vi "Sequence setup GUI.vi"(11 "error in (no error)":errorcluster) -> (8 "OK":bool, 15 "error out":errorcluster)   [LabVIEW 2011]
uses:
  Sequence step GUI.ctl
  X-cont Action select/Action select.xctl
  X-cont criteria/Criteria control.xctl
  Boolean operation.ctl
  User input.ctl
  Complete sequence cluster holder.ctl
  Sequence steps config..ctl
  Single criteria cluster.ctl
  Criteria types.ctl
panel:
  in  "User input 1":T1={"Input name"="", "Minimum value "=-inf, "Maximum value"=inf, "Default value"=0.0, "User inp enabled"=FALSE}
  in  "Move up":bool
  in  "Move down":bool
  in  "Sequences":i32(listbox)
  in  "Delete step":bool
  in  "Add step":bool
  in  "Delete sequence":bool
  in  "New sequence":bool
  in  "Step":T2
  in  "Steps":i32(listbox)
  out "Mode":bool
  in  "Help":bool
  in  "Done":bool
  # "User input"
  # "Tab header s can be changed as wanted\n\nCustom can be used for completly ccutom behavior,\nmust then highjack  an other hidden page, for settings"
  # "Add custom behavior taht cvan not be replicated by a simple cluster with valisdity checking"
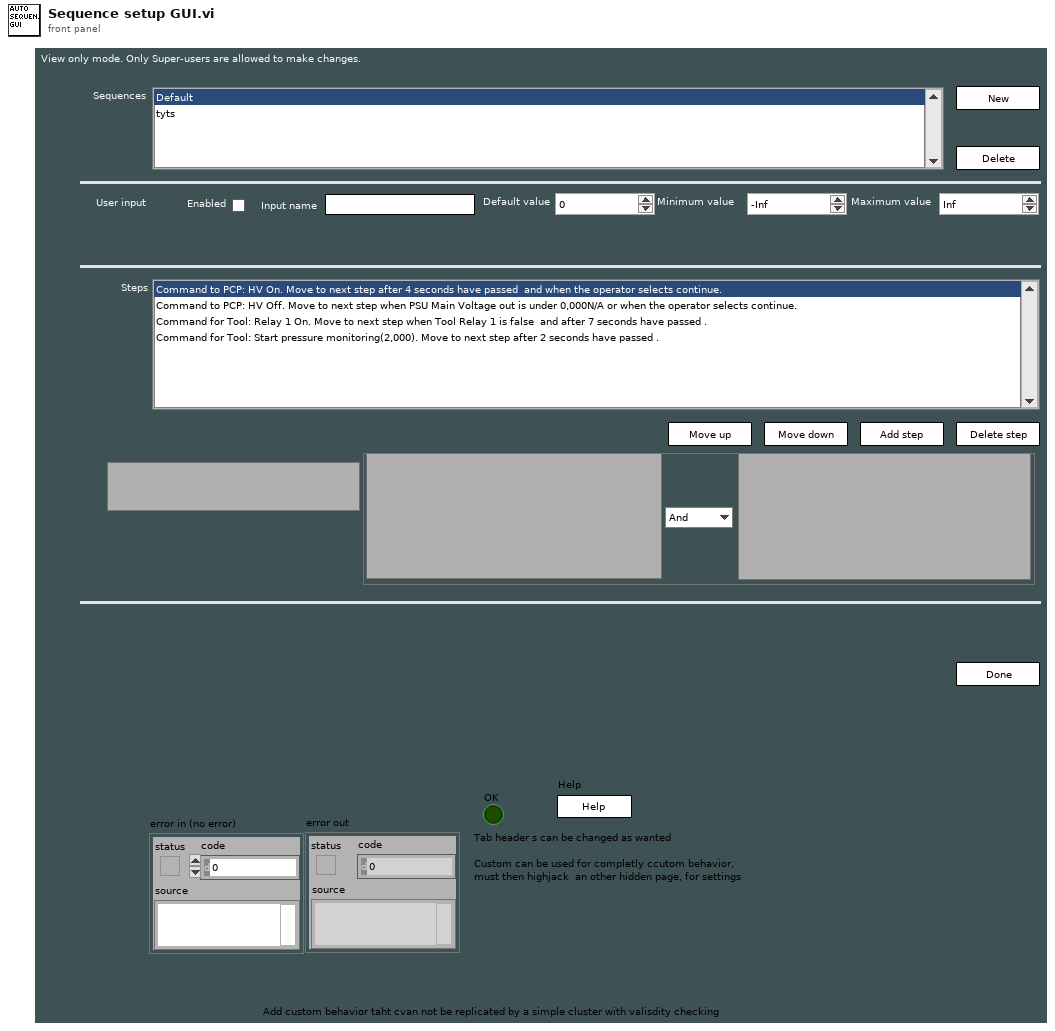
[diagram p1: front panel]
types:
  T1 = typedef "User input.ctl" = cluster{"Input name":string, "Minimum value ":dbl, "Maximum value":dbl, "Default value":dbl, "User inp enabled":bool}
  T2 = typedef "Sequence step GUI.ctl" = cluster{"Action select":cluster{"Action index":i32, "Data":dbl}, "Criteria 1":cluster{"Criteria":T3}, "C1 op C2":T5, "Criteria 2":cluster{"Criteria":T3}}
  T3 = typedef "Single criteria cluster.ctl" = cluster{"Criteria":T4, "Time or analog value":dbl, "Primary IO index":i32, "Secondary  IO index":i32, "User_input":bool}
  T4 = typedef "Criteria types.ctl" = enum16{"No criteria(True)", "Time(s)", "Analog IO over", "Analog IO over or equal", "Analog IO under", "Analog IO under or equal", "Analog IO 1 minus Analog IO 2 over", "Digital IO True", "Digital IO False", "Operator approval"}
  T5 = typedef "Boolean operation.ctl" = enum16{"And", "Or", "Xor", "Nand", "Nor", "Nxor", "Implies"}
  T6 = enum16{"GET", "SET", "Get from Ini", "Put in Ini"}
  T7 = typedef "User Indikator.ctl" = cluster{"User Name":string, "Super User":T8}
  T8 = typedef "Super User bool indikator.ctl" = bool
  T9 = enum8{"Enabled", "Disabled", "Disabled and Grayed Out"}
  T10 = typedef "Sequence steps config..ctl" = cluster{"Enabled":bool, "Criteria 1":T3, "C1 op C2":T5, "Criteria 2":T3, "Action index":i32, "Action Name":string, "Action value":dbl}
  T11 = typedef "Fixed Analog Channel Definition.ctl" = cluster{"ID":u16, "Name":string, "Quantity":T12, "Unit":string, "Maximum upd":T13, "Comment":string, "Help file Name":string, "Help file Section ":string, "Category":T14, "User adjustable Scaling":bool, "Default Scaling":T15, "Default Unit":i32, "Classification":T16}
  T12 = typedef "Quantity enum.ctl" = enum16{"NA", "Acceleration", "Angle", "Current", "Force", "Distance", "Pressure", "Resistance", "Rotational Speed", "Speed", "Temperature", "Tension", "Torque", "Voltage", "Weight"}
  T13 = typedef "Update frequensies.ctl" = enum16{"2 Hz", "1 Hz", "0.1 Hz"}
  T14 = typedef "Channel catagory Enum.ctl" = enum16{"No Category", "Power", "Temperature", "Pressure"}
  T15 = typedef "Scaling.ctl" = cluster{"Gain":dbl, "Offset":dbl}
  T16 = typedef "Channel Classification Enum.ctl" = enum16{"Basic", "Advanced", "Expert", "Unused"}
  T17 = typedef "Fixed Digital Channel Definition.ctl" = cluster{"ID":u16, "Name":string, "NA Text":string, "Off Text":string, "On Text":string, "Maximum upd":T13, "Comment":string, "Help file Name":string, "Help file Section ":string, "Catagory":T14, "In use":bool}
  T18 = typedef "Analog Var Disp 0 sif.ctl" = cluster{"Value":dbl, "Unit":string, "Status":T19}
  T19 = typedef "Status indicator Black Small.ctl" = u16
  T20 = typedef "Action colleciton cluster.ctl" = cluster{"common":T21, "Action type":T23, "General command":T24, "PCP command":T25, "Tool command":T26}
  T21 = typedef "Action common elements.ctl" = cluster{"Name":string, "Adjuster type":T22, "Adjuster double default value":dbl}
  T22 = typedef "Action adjuster type.ctl" = enum16{"Non", "Double"}
  T23 = typedef "Action type.ctl" = enum16{"General", "PCP command", "Tool command"}
  T24 = typedef "General command list.ctl" = enum16{"No action"}
  T25 = typedef "PCP High Level Commands.ctl" = enum16{"HVPSU HV ON", "HVPSU HV OFF", "PCP PC", "PCP Local", "Update Motor Voltage", "Update Cable Resistance", "Final Motor Voltage", "Final Resistance"}
  T26 = typedef "Tool specific commands.ctl" = enum16{"controller relay 1 on", "controller relay 1 off", "controller relay 2 on", "controller relay 2 off", "Solonoid 1 (master) on", "Solonoid 1 (master) off", "Solonoid 2 (Stroker) on", "Solonoid 2 (Stroker) off", "Solonoid 3 (Anchor) on", "Solonoid 3 (Anchor) off", "Controller relay 1 & 2 on", "Controller relay 1 & 2 off", "Controller relay 1 on, 2 off", "Controller relay 1 off, 2 on", "STROKER tool: Stop Force Mon", "High-G Stop", "High-G Get data", "High-G Stop Get data", "STROKER tool: Stroke out", "STROKER tool: Stroke in", "STROKER tool: Stroke stop", "STROKER tool: Stroke go to", "STROKER tool: Stop Homing", "STROKER tool: Start Force Mon dir in", "STROKER tool: Start Force Mon dir out", "Controller STOP"}
  T27 = typedef "Complete sequence cluster holder.ctl" = cluster{"Sequence Name":string, "User input 1":T1, "Steps":T10[]}
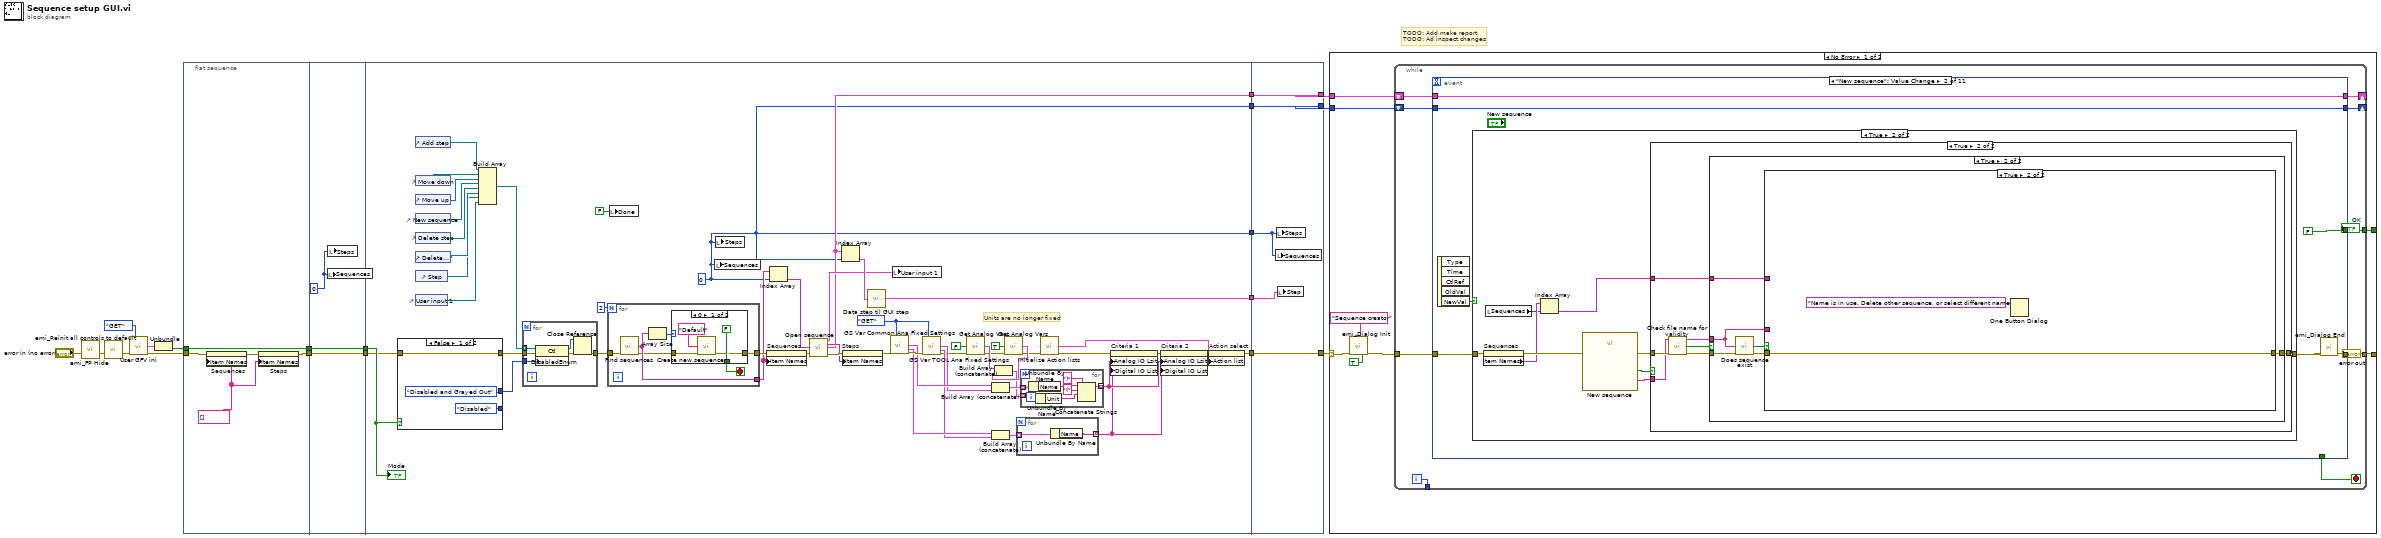
[diagram p0: block diagram]
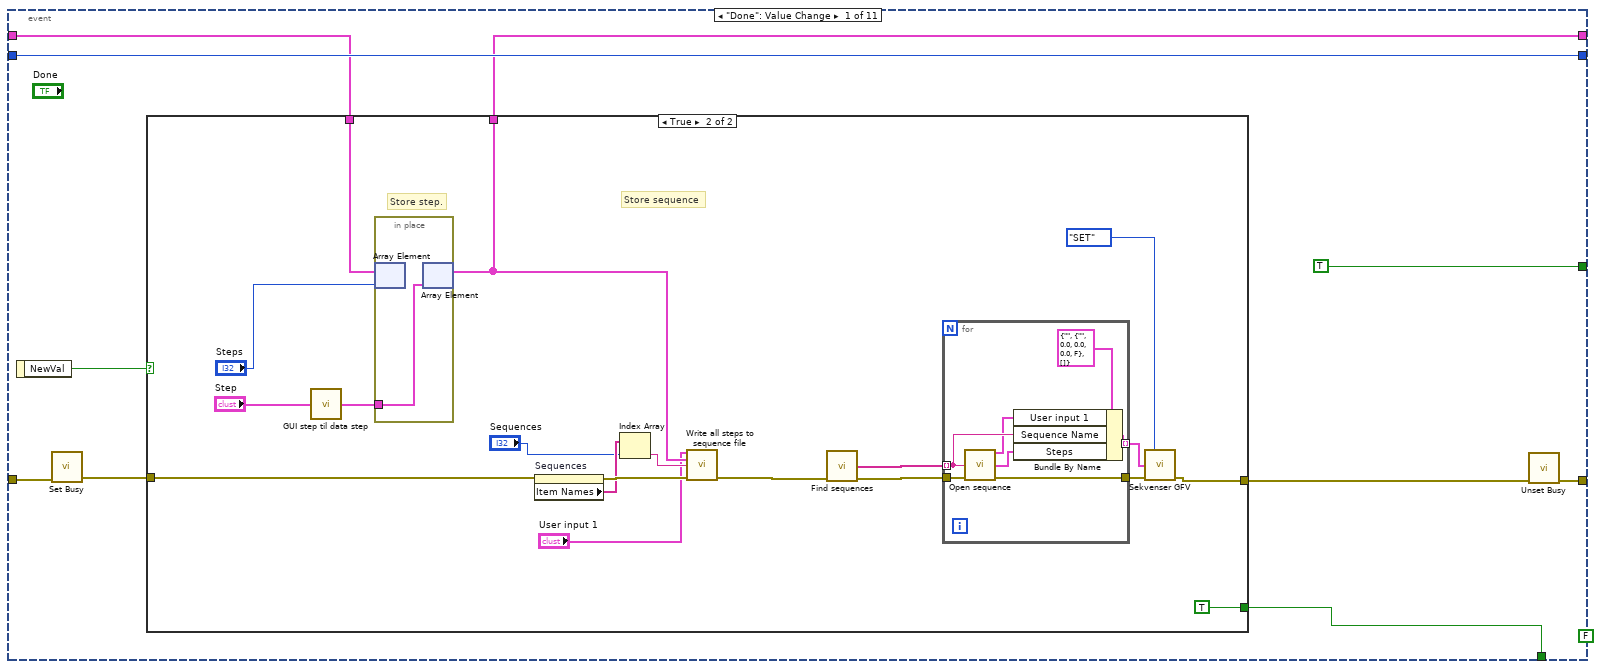
[diagram p2: hidden frame]
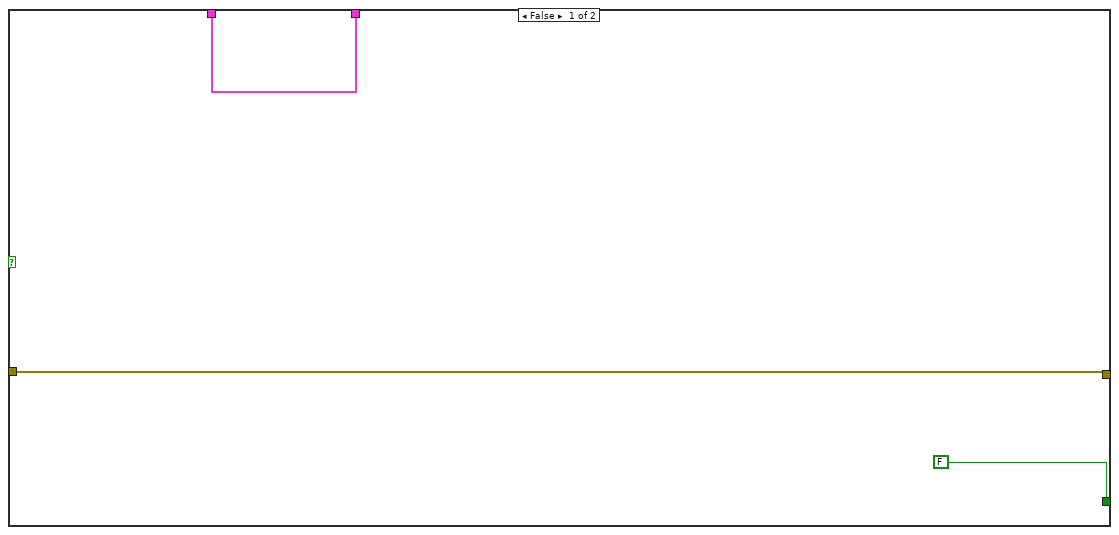
[diagram p3: hidden frame]
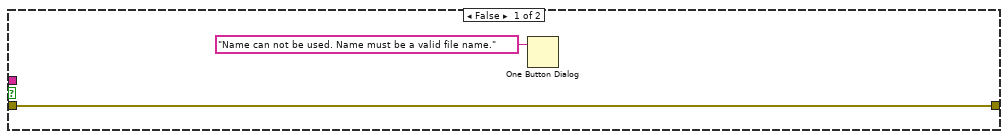
[diagram p6: hidden frame]
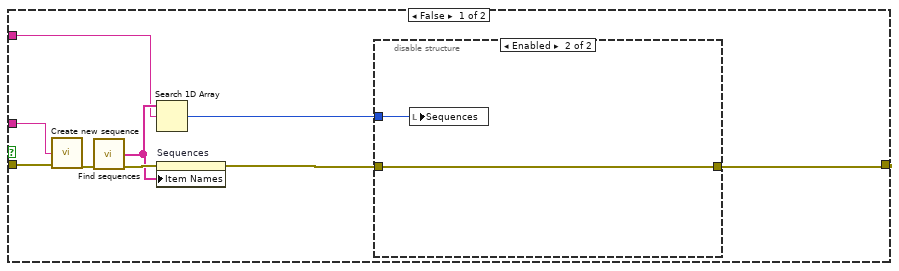
[diagram p7: hidden frame]
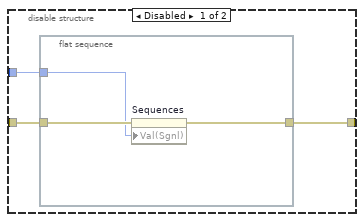
[diagram p8: hidden frame]
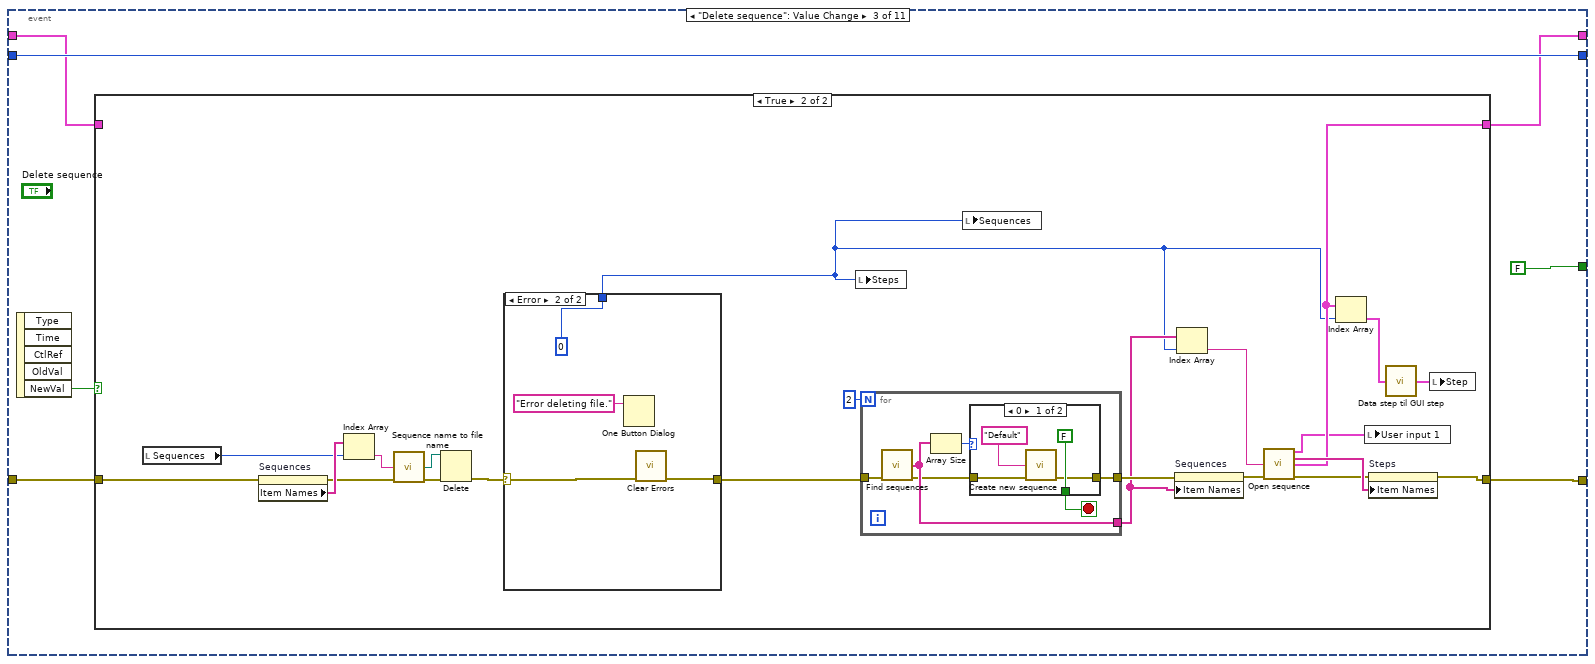
[diagram p9: hidden frame]
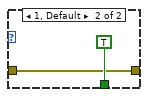
[diagram p11: hidden frame]
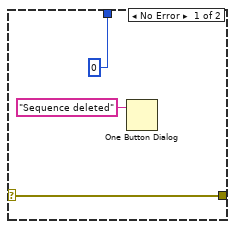
[diagram p12: hidden frame]
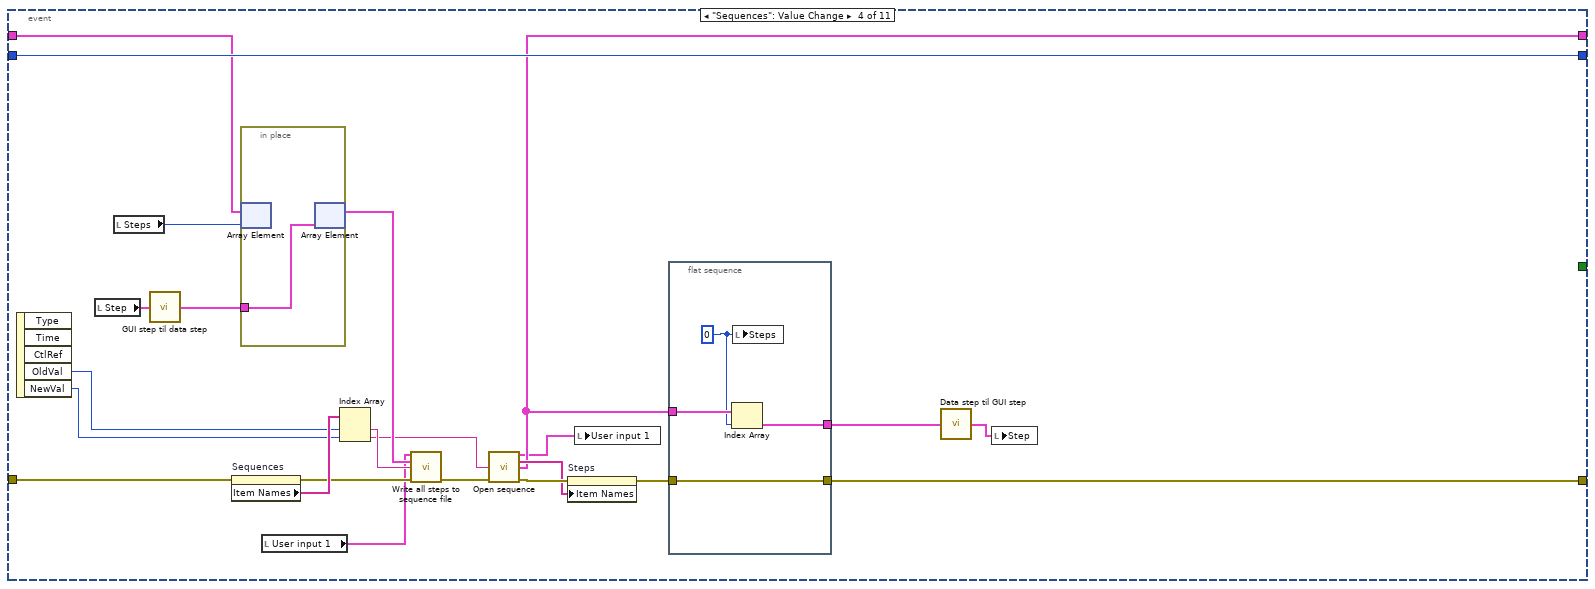
[diagram p13: hidden frame]
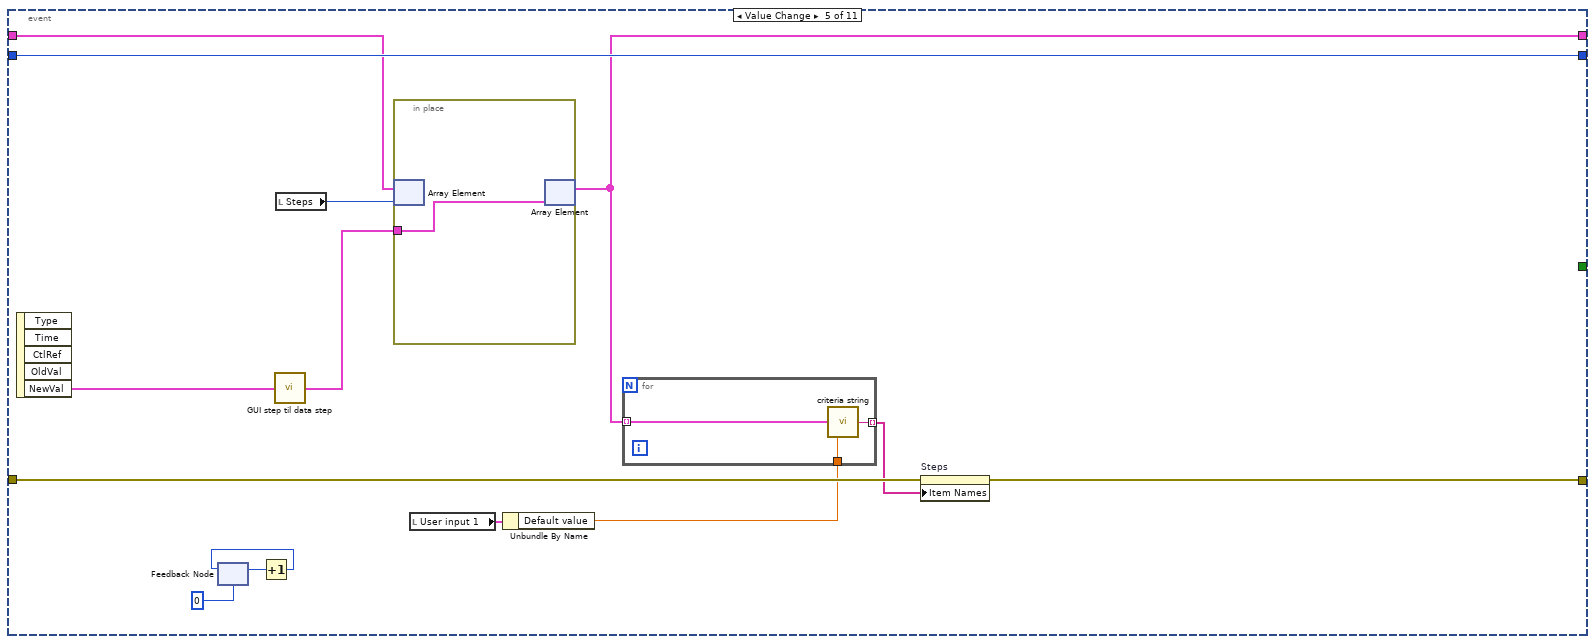
[diagram p14: hidden frame]
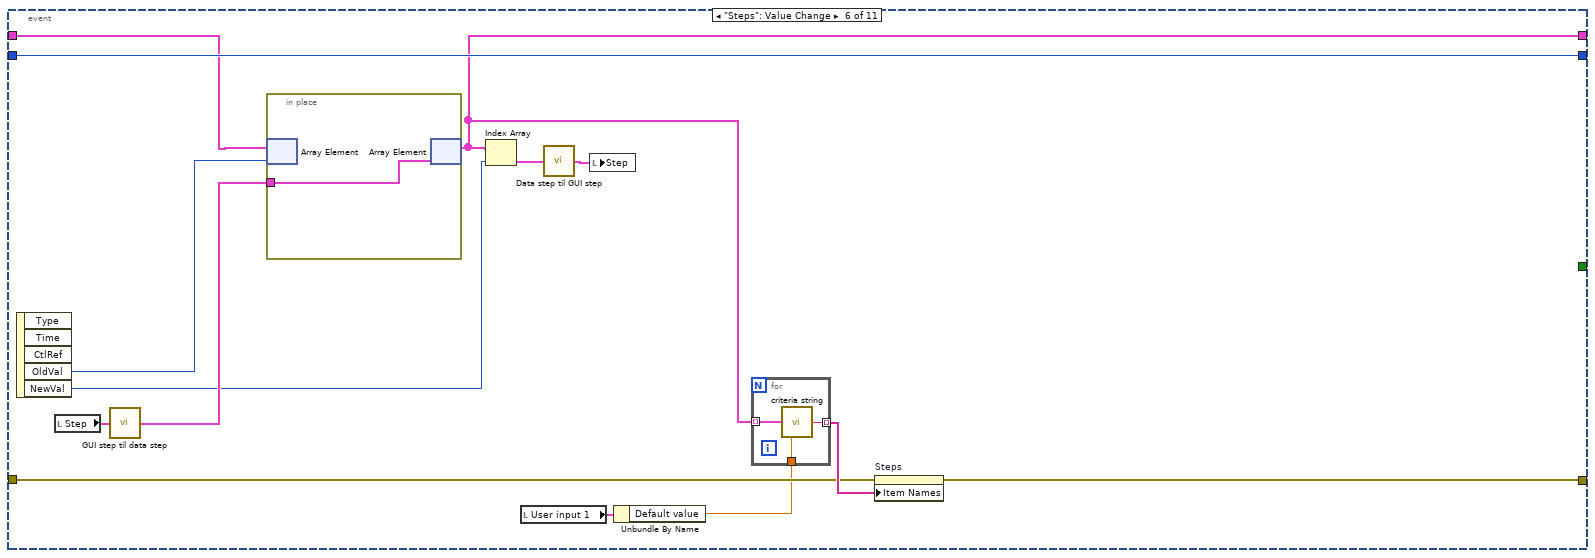
[diagram p15: hidden frame]
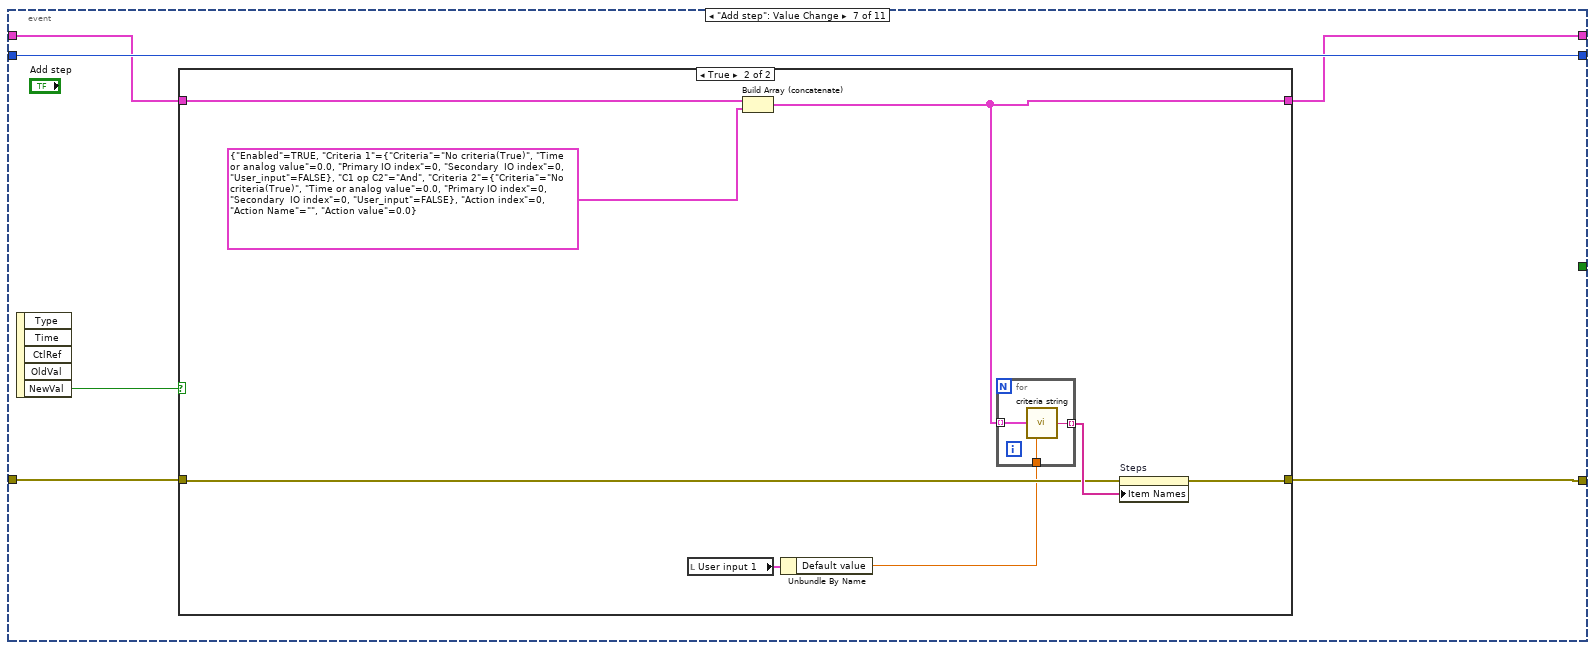
[diagram p16: hidden frame]
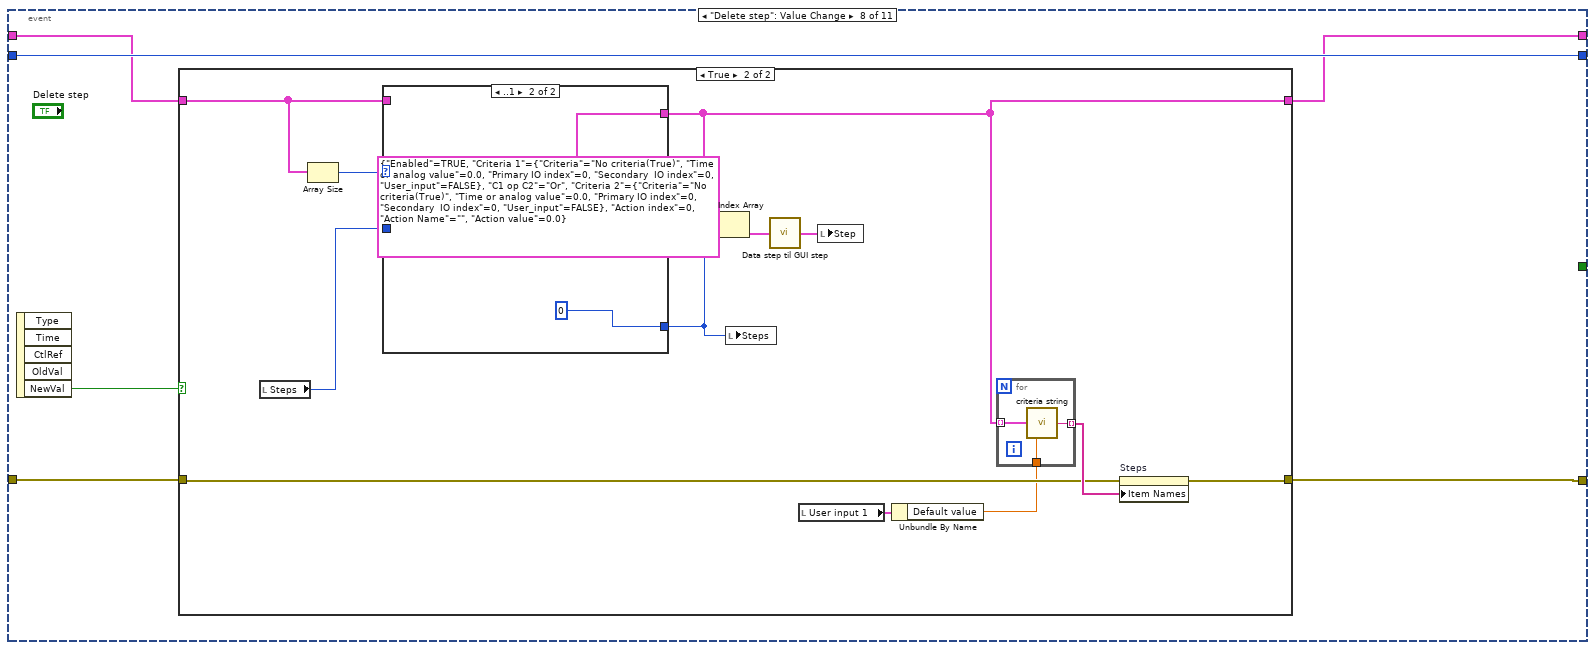
[diagram p18: hidden frame]
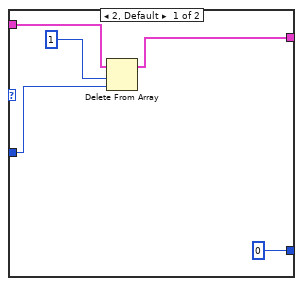
[diagram p20: hidden frame]
diagram:
  # "TODO: Add make report\nTODO: Ad inspect changes"
  n1 = call "emi_FP Hide.vi"("error in (no error)"="error in (no error)") -> ("error out"=w18:errorcluster)  [unwired: 13 in, 1 out]
  n2 = call "emi_Reinit all controls to default.vi"("error in (no error)"=w18) -> ("error out"=w16:errorcluster)  [unwired: 13 in, 1 out]
  n3 = call "User GFV ini.vi"("Action(GET)"=T6."GET", "error in (no error)"=w16) -> ("User ID out"=w15:T7, "error out"=w14:errorcluster)  [unwired: 12 in]
  n4 = Unbundle(w15) -> ("Super User"=w13:T8)  [unwired: 1 out]
  n5 = flat-sequence {
    tunnel: w13 -> [w27]
    tunnel: w14 -> [w26]
    tunnel: [w23] -> w9
    tunnel: [w27] -> w7
    tunnel: w9 -> [w30]
    tunnel: [w30] -> w8
    tunnel: w7 -> [w29]
    tunnel: [w29] -> w6
    tunnel: w8 -> [w80]
    tunnel: w6 -> [w81]
    tunnel: [w47] -> w5
    tunnel: [w42] -> w4
    tunnel: [w41] -> w3
    tunnel: [w41] -> w2
    tunnel: [w40] -> w1
    tunnel: [w116] -> w10
    tunnel: [w117] -> w11
    tunnel: [w118] -> w17
    tunnel: w5 -> [w118]
    tunnel: w4 -> [w117]
    tunnel: w3 -> [w116]
    tunnel: w2 -> [w115]
    tunnel: w1 -> [w114]
    frame #0 {
      w24 = string[] [] ("Item Names")
      n6 = property on="Sequences" class="LstBox (strict)"(error in=w26, "Item Names"=w24) -> (error out=w25:errorcluster)  [unwired: 1 in, 1 out]
      n7 = property on="Steps" class="LstBox (strict)"(error in=w25, "Item Names"=w24) -> (error out=w23:errorcluster)  [unwired: 1 in, 1 out]
    }
    frame #1 {
      w28 = 0 ("Sequences")
      n8 = local write "Sequences"(w28) -> ()
      n9 = local write "Steps"(w28) -> ()
    }
    frame #2 {
      w59 = enum16{"GET", "SET"}."GET" ("Action(GET)")
      w41 = 0 ("Sequences")
      # "Units are no longer fixed"
      n10 = case shown="False" w81 {
        tunnel: w80 -> [w110 w113]
        tunnel: [w110 w113] -> w65
        tunnel: [T9."Disabled and Grayed Out" ("Disabled") w112] -> w61
        tunnel: [T9."Disabled" ("Disabled") w112] -> _
        frame False {
        }
        frame True {
          w112 = T9."Enabled" ("Disabled")
        }
      }
      n11 = control-ref of="Add step"() -> (w66:refnum<vi>)
      n12 = control-ref of="Move down"() -> (w67:refnum<vi>)
      n13 = control-ref of="Move up"() -> (w68:refnum<vi>)
      n14 = control-ref of="New sequence"() -> (w69:refnum<vi>)
      n15 = control-ref of="Delete step"() -> (w70:refnum<vi>)
      n16 = control-ref of="Delete sequence"() -> (w71:refnum<vi>)
      n17 = control-ref of="Step"() -> (w62:refnum<vi>)
      n18 = control-ref of="User input 1"() -> (w43:refnum<vi>)
      n19 = Build Array(w66, w67, w68, w69, w70, w71, w62, w43) -> (w63:refnum<vi>[])
      n20 = for {
        tunnel: w65 -> [w96]
        tunnel: [w94] -> w64
        tunnel: w63 -> [w92] mode=indexing
        tunnel: w61 -> [w91]
        n21 = property class="Ctl"(reference=w92, error in=w96, "DisabledEnum"=w91) -> (reference out=w93:refnum<vi>, error out=w95:errorcluster)
        n22 = Close Reference(reference=w93, error in (no error)=w95) -> (error out=w94:errorcluster)
      }
      n23 = for {
        N: 2 -> [_]
        tunnel: w64 -> [w102]
        tunnel: [w97] -> w79
        tunnel: [w101] -> w77
        stop <- w98 stop-if-true
        n24 = call "Find sequences.vi"("error in (no error)"=w102) -> ("Sequences"=w101:string[], "error out"=w100:errorcluster)  [unwired: 13 in]
        n25 = Array Size(array=w101) -> (size(s)=w99:i32)
        n26 = case shown="0" w99 {
          tunnel: w100 -> [w105 w107]
          tunnel: [FALSE TRUE] -> w98
          tunnel: [w104 w107] -> w97
          frame 0 {
            n27 = call "Create new sequence.vi"("Sequence name"="Default", "error in (no error)"=w105) -> ("error out"=w104:errorcluster)  [unwired: 13 in]
          }
          frame 1, Default {
          }
        }
      }
      n28 = local write "Done"(FALSE ("Done")) -> ()
      n29 = local write "Sequences"(w41) -> ()
      n30 = local write "Steps"(w41) -> ()
      n31 = property on="Sequences" class="LstBox (strict)"(error in=w79, "Item Names"=w77) -> (error out=w76:errorcluster)  [unwired: 1 in, 1 out]
      n32 = Index Array(array=w77, index=w41) -> (element=w75:string)
      n33 = call "Open sequence.vi"("Sequence name"=w75, "error in (no error)"=w76) -> ("User input 1"=w44:T1, "string steps"=w73:string[], "Steps"=w42:T10[], "error out"=w74:errorcluster)  [unwired: 9 in, 1 out]
      n34 = Index Array(array=w42, index=w41) -> (element=w72:T10)
      n35 = property on="Steps" class="LstBox (strict)"(error in=w74, "Item Names"=w73) -> (error out=w52:errorcluster)  [unwired: 1 in, 1 out]
      n36 = call "Data step til GUI step.vi"("data step cluster"=w72) -> ("GUI step clluster"=w40:T2)  [unwired: 13 in, 1 out]
      n37 = call "GS Var Common Ana Fixed Settings.vi"("Action(GET)"=w59, "error in (no error)"=w52) -> ("Common Analog Var Fixed out"=w58:T11[], "Common Digital var Fixed"=w56:T17[], "error out"=w60:errorcluster)  [unwired: 11 in]
      n38 = local write "User input 1"(w44) -> ()
      n39 = call "GS Var TOOL Ana Fixed Settings.vi"("Action(GET)"=w59, "error in (no error)"=w60) -> ("Tool Analog var Fixed out"=w57:T11[], "Tool Digital Var Fixed out"=w55:T17[], "error out"=w34:errorcluster)  [unwired: 11 in]
      n40 = call "Get Analog Vars.vi"("Tool"=FALSE, "error in (no error)"=w34) -> ("Analog Vars"=w38:T18[], "error out"=w37:errorcluster)  [unwired: 7 in, 5 out]
      n41 = Build Array (concatenate)(w58, w57) -> (w54:T11[])
      n42 = Build Array (concatenate)(w56, w55) -> (w53:T17[])
      n43 = call "Get Analog Vars.vi"("Tool"=TRUE, "error in (no error)"=w37) -> ("Analog Vars"=w39:T18[], "error out"=w33:errorcluster)  [unwired: 7 in, 5 out]
      n44 = Build Array (concatenate)(w38, w39) -> (w31:T18[])
      n45 = for {
        tunnel: w53 -> [w83] mode=indexing
        tunnel: [w82] -> w49 mode=indexing
        n46 = Unbundle By Name(w83) -> ("Name"=w82:string)
      }
      n47 = for {
        tunnel: w54 -> [w90] mode=indexing
        tunnel: [w88] -> w50 mode=indexing
        tunnel: w31 -> [w85] mode=indexing
        n48 = Unbundle By Name(w90) -> ("Name"=w89:string)
        n49 = Unbundle By Name(w85) -> ("Unit"=w84:string)
        n50 = Concatenate Strings(w89, "(" ("string"), w84, ")" ("string")) -> (w88:string)
      }
      n51 = call "Initialize Action lists.vi"("error in (no error)"=w33) -> ("Actions"=w32:T20[], "error out"=w46:errorcluster)  [unwired: 12 in, 1 out]
      n52 = property on="Criteria 1" class="Criteria control (strict)"(error in=w46, "Analog IO Lsit"=w50, "Digital IO List"=w49) -> (error out=w51:errorcluster)  [unwired: 1 in, 1 out]
      n53 = property on="Criteria 2" class="Criteria control (strict)"(error in=w51, "Analog IO Lsit"=w50, "Digital IO List"=w49) -> (error out=w48:errorcluster)  [unwired: 1 in, 1 out]
      n54 = property on="Action select" class="Action select (strict)"(error in=w48, "Action list"=w32) -> (error out=w47:errorcluster)  [unwired: 1 in, 1 out]
      "Mode" <- w81
    }
    frame #3 {
      n55 = local write "Sequences"(w115) -> ()
      n56 = local write "Steps"(w115) -> ()
      n57 = local write "Step"(w114) -> ()
    }
  }
  n58 = case shown="No Error" w17 {
    selector: w17 -> [w122 w467]
    tunnel: [w121 FALSE] -> w21
    tunnel: [w126 w467] -> w20
    tunnel: w11 -> [w120 _]
    tunnel: w10 -> [w119 _]
    frame No Error {
      n59 = call "emi_Dialog Init.vi"("Header String(\"\")"="Sequence creator" ("Header String(\"\")"), "error in"=w122, "Modal(T)"=TRUE) -> ("error out"=w125:errorcluster)  [unwired: 12 in]
      n60 = while {
        tunnel: [w135] -> _
        tunnel: w125 -> [w133]
        tunnel: [w132] -> w126
        tunnel: [w131] -> w121
        shift-right: [w129] -> _
        shift-left: w120 -> [w130]
        shift-right: [w127] -> _
        shift-left: w119 -> [w128]
        i -> [w135]
        stop <- w134 stop-if-true
        n61 = event shown="[1] \"New sequence\": Value Change" {
          selector: _ -> [_ _ _ _ _ _ _ _ _ _ _]
          dyn-events: _ -> [_ _ _ _ _ _ _ _ _ _ _]
          timeout: _ -> [_ _ _ _ _ _ _ _ _ _ _]
          tunnel: [w136 _ _ _ _ _ _ _ _ _ FALSE] -> w134
          tunnel: w133 -> [w141 w178 w230 w294 w313 w327 w344 w363 w394 w424 w456]
          tunnel: [w139 w179 w231 w279 w312 w325 w343 w362 w393 w423 w457] -> w132
          tunnel: [TRUE FALSE FALSE _ _ _ _ _ _ _ _] -> w131
          tunnel: w130 -> [w143 w176 w228 w295 w317 w332 w342 w361 w392 w422 w454]
          tunnel: [w142 w176 w227 w281 w311 w326 w341 w360 w391 w421 w454] -> w129
          tunnel: w128 -> [w144 w180 w232 w299 w318 w336 w346 w365 w396 w426 w453]
          tunnel: [w144 w180 w232 w299 w318 w336 w346 w365 w396 w426 w453] -> w127
          event "Done": Value Change {
            (unwired) FALSE
            (unwired) FALSE
            n62 = event-data() -> ("NewVal"=w137:bool)  [unwired: 1 in]
            n63 = call <vilib>:"Set Busy.vi"("error in (no error)"=w141) -> ("error out"=w140:errorcluster)  [unwired: 9 in, 1 out]
            n64 = case shown="True" w137 {
              tunnel: w143 -> [w147 w167]
              tunnel: [w147 w159] -> w142
              tunnel: w140 -> [w148 w154]
              tunnel: [w148 w152] -> w138
              tunnel: [FALSE TRUE] -> w136
              frame False {
              }
              frame True {
                # "Store sequence"
                # "Store step."
                n65 = call "GUI step til data step.vi"("GUI step clluster"="Step") -> ("data step cluster"=w164:T10)  [unwired: 14 in]
                n66 = in-place {
                  in-place-border: w164 -> [w175]
                  n67 = in-place-array #1(w167, "Steps") -> ()  [unwired: 1 out]
                  n68 = in-place-array #1(w175) -> (w159:T10[])  [unwired: 1 out]
                }
                n69 = property on="Sequences" class="LstBox (strict)"(error in=w154) -> (error out=w163:errorcluster, "Item Names"=w162:string[])  [unwired: 1 in, 1 out]
                n70 = Index Array(array=w162, index="Sequences") -> (element=w160:string)
                n71 = call "Write all steps to sequence file.vi"("User input 1"="User input 1", "Sequence"=w159, "Sequence name"=w160, "error in (no error)"=w163) -> ("error out"=w153:errorcluster)  [unwired: 11 in]
                n72 = call "Find sequences.vi"("error in (no error)"=w153) -> ("Sequences"=w156:string[], "error out"=w157:errorcluster)  [unwired: 13 in]
                n73 = for {
                  tunnel: [w173] -> w158
                  tunnel: w157 -> [w174]
                  tunnel: w156 -> [w170] mode=indexing
                  tunnel: [w169] -> w155 mode=indexing
                  n74 = call "Open sequence.vi"("Sequence name"=w170, "error in (no error)"=w174) -> ("User input 1"=w168:T1, "Steps"=w171:T10[], "error out"=w173:errorcluster)  [unwired: 9 in, 2 out]
                  n75 = Bundle By Name(cluster=T27 {"Sequence Name"="", "User input 1"={"Input name"="", "Minimum value "=0.0, "Maximum value"=0.0, "Default value"=0.0, "User inp enabled"=FALSE}, "Steps"=[]} ("Sequence in"), "User input 1"=w168, "Sequence Name"=w170, "Steps"=w171) -> (w169:T27)
                }
                n76 = call "Sekvenser GFV.vi"("Action(GET)"=enum16{"GET", "SET"}."SET", "Sequences"=w155, "error in (no error)"=w158) -> ("error out"=w152:errorcluster)  [unwired: 11 in, 1 out]
              }
            }
            n77 = call <vilib>:"Unset Busy.vi"("error in (no error)"=w138) -> ("error out"=w139:errorcluster)  [unwired: 10 in]
          }
          event "New sequence": Value Change {
            n78 = event-data() -> ("NewVal"=w177:bool)  [unwired: 1 in, 4 out]
            n79 = case shown="True" w177 {
              tunnel: [w182 w189] -> w179
              tunnel: w178 -> [w182 w187]
              frame False {
              }
              frame True {
                n80 = property on="Sequences" class="LstBox (strict)"(error in=w187) -> (error out=w186:errorcluster, "Item Names"=w185:string[])  [unwired: 1 in, 1 out]
                n81 = local read "Sequences"() -> (w184:i32)
                n82 = Index Array(array=w185, index=w184) -> (element=w183:string)
                n83 = call "New sequence"("error in (no error)"=w186) -> ("Name"=w188:string, "OK"=w191:bool, "error out"=w190:errorcluster)  [unwired: 16 in]
                n84 = case shown="True" w191 {
                  tunnel: w190 -> [w192 w199]
                  tunnel: [w192 w197] -> w189
                  tunnel: w188 -> [_ w198]
                  tunnel: w183 -> [_ w193]
                  frame False {
                  }
                  frame True {
                    n85 = call "Check file name for validity.vi"("String in"=w198, "error in (no error)"=w199) -> ("String out"=w194:string, "Valid File of folder name"=w195:bool, "error out"=w196:errorcluster)  [unwired: 11 in]
                    n86 = case shown="True" w195 {
                      tunnel: [w201 w206] -> w197
                      tunnel: w196 -> [w201 w207]
                      tunnel: w194 -> [_ w203]
                      tunnel: w193 -> [_ w202]
                      frame False {
                        n87 = One Button Dialog(message="Name can not be used. Name must be a valid file name.") -> ()  [unwired: 1 in, 1 out]
                      }
                      frame True {
                        n88 = call "Does sequence exist.vi"("Sequence name"=w203, "error in (no error)"=w207) -> ("Sequence  exsists"=w204:bool, "error out"=w205:errorcluster)  [unwired: 12 in]
                        n89 = case shown="True" w204 {
                          tunnel: [w211 w226] -> w206
                          tunnel: w205 -> [w216 w226]
                          tunnel: w203 -> [w212 _]
                          tunnel: w202 -> [w208 _]
                          frame False {
                            n90 = call "Create new sequence.vi"("Sequence name"=w212, "error in (no error)"=w216) -> ("error out"=w215:errorcluster)  [unwired: 13 in]
                            n91 = call "Find sequences.vi"("error in (no error)"=w215) -> ("Sequences"=w213:string[], "error out"=w214:errorcluster)  [unwired: 13 in]
                            n92 = Search 1D Array(1D array=w213, element=w208) -> (index of element=w209:i32)  [unwired: 1 in]
                            n93 = property on="Sequences" class="LstBox (strict)"(error in=w214, "Item Names"=w213) -> (error out=w210:errorcluster)  [unwired: 1 in, 1 out]
                            n94 = disable-structure shown="Enabled" {
                              disable-tunnel: [w219 w224] -> w211
                              disable-tunnel: w210 -> [w218 w224]
                              disable-tunnel: w209 -> [w217 w223]
                              frame Disabled {
                                n95 = flat-sequence {
                                tunnel: [w221] -> w219
                                tunnel: w218 -> [w222]
                                tunnel: w217 -> [w220]
                                frame #0 {
                                n96 = property on="Sequences" class="LstBox (strict)"(error in=w222, "Val(Sgnl)"=w220) -> (error out=w221:errorcluster)  [unwired: 1 in, 1 out]
                                }
                                }
                              }
                              frame Enabled {
                                n97 = local write "Sequences"(w223) -> ()
                              }
                            }
                          }
                          frame True {
                            n98 = One Button Dialog(message="Name is in use. Delete other sequence, or select different name.") -> ()  [unwired: 1 in, 1 out]
                          }
                        }
                      }
                    }
                  }
                }
              }
            }
          }
          event "Delete sequence": Value Change {
            n99 = event-data() -> ("NewVal"=w229:bool)  [unwired: 1 in, 4 out]
            n100 = case shown="True" w229 {
              tunnel: [w235 w243] -> w231
              tunnel: w230 -> [w235 w256]
              tunnel: w228 -> [w234 _]
              tunnel: [w234 w239] -> w227
              frame False {
              }
              frame True {
                n101 = local read "Sequences"() -> (w254:i32)
                n102 = property on="Sequences" class="LstBox (strict)"(error in=w256) -> (error out=w255:errorcluster, "Item Names"=w257:string[])  [unwired: 1 in, 1 out]
                n103 = Index Array(array=w257, index=w254) -> (element=w238:string)
                n104 = call "Sequence name to file name.vi"("Sequence name"=w238, "error in (no error)"=w255) -> ("Sequence file path"=w252:path, "error out"=w253:errorcluster)  [unwired: 12 in]
                n105 = Delete(path (use dialog)=w252, error in=w253) -> (error out=w251:errorcluster)  [unwired: 3 in, 2 out]
                n106 = case shown="Error" w251 {
                  selector: w251 -> [w271 w276]
                  tunnel: [w271 w275] -> w249
                  tunnel: [0 ("Sequences") 0 ("Sequences")] -> w237
                  frame No Error {
                    n107 = One Button Dialog(message="Sequence deleted") -> ()  [unwired: 1 in, 1 out]
                  }
                  frame Error {
                    n108 = One Button Dialog(message="Error deleting file.") -> ()  [unwired: 1 in, 1 out]
                    n109 = call <vilib>:"Clear Errors.vi"("error in (no error)"=w276) -> ("error out"=w275:errorcluster)  [unwired: 6 in]
                  }
                }
                n110 = local write "Steps"(w237) -> ()
                n111 = for {
                  N: 2 -> [_]
                  tunnel: w249 -> [w263]
                  tunnel: [w258] -> w244
                  tunnel: [w262] -> w242
                  stop <- w259 stop-if-true
                  n112 = call "Find sequences.vi"("error in (no error)"=w263) -> ("Sequences"=w262:string[], "error out"=w261:errorcluster)  [unwired: 13 in]
                  n113 = Array Size(array=w262) -> (size(s)=w260:i32)
                  n114 = case shown="0" w260 {
                    tunnel: w261 -> [w266 w268]
                    tunnel: [FALSE TRUE] -> w259
                    tunnel: [w265 w268] -> w258
                    frame 0 {
                      n115 = call "Create new sequence.vi"("Sequence name"="Default", "error in (no error)"=w266) -> ("error out"=w265:errorcluster)  [unwired: 13 in]
                    }
                    frame 1, Default {
                    }
                  }
                }
                n116 = local write "Sequences"(w237) -> ()
                n117 = property on="Sequences" class="LstBox (strict)"(error in=w244, "Item Names"=w242) -> (error out=w245:errorcluster)  [unwired: 1 in, 1 out]
                n118 = Index Array(array=w242, index=w237) -> (element=w246:string)
                n119 = call "Open sequence.vi"("Sequence name"=w246, "error in (no error)"=w245) -> ("User input 1"=w236:T1, "string steps"=w248:string[], "Steps"=w239:T10[], "error out"=w247:errorcluster)  [unwired: 9 in, 1 out]
                n120 = Index Array(array=w239, index=w237) -> (element=w240:T10)
                n121 = local write "User input 1"(w236) -> ()
                n122 = property on="Steps" class="LstBox (strict)"(error in=w247, "Item Names"=w248) -> (error out=w243:errorcluster)  [unwired: 1 in, 1 out]
                n123 = call "Data step til GUI step.vi"("data step cluster"=w240) -> ("GUI step clluster"=w241:T2)  [unwired: 13 in, 1 out]
                n124 = local write "Step"(w241) -> ()
              }
            }
          }
          event "Sequences": Value Change {
            n125 = event-data() -> ("OldVal"=w292:i32, "NewVal"=w291:i32)  [unwired: 1 in, 3 out]
            n126 = local read "Step"() -> (w298:T2)
            n127 = local read "Steps"() -> (w297:i32)
            n128 = call "GUI step til data step.vi"("GUI step clluster"=w298) -> ("data step cluster"=w296:T10)  [unwired: 14 in]
            n129 = property on="Sequences" class="LstBox (strict)"(error in=w294) -> (error out=w290:errorcluster, "Item Names"=w293:string[])  [unwired: 1 in, 1 out]
            n130 = in-place {
              in-place-border: w296 -> [w304]
              n131 = in-place-array #2(w295, w297) -> ()  [unwired: 1 out]
              n132 = in-place-array #2(w304) -> (w288:T10[])  [unwired: 1 out]
            }
            n133 = local read "User input 1"() -> (w278:T1)
            n134 = Index Array(array=w293, index #1=w292, index #2=w291) -> (element #1=w289:string, element #2=w286:string)
            n135 = call "Write all steps to sequence file.vi"("User input 1"=w278, "Sequence"=w288, "Sequence name"=w289, "error in (no error)"=w290) -> ("error out"=w287:errorcluster)  [unwired: 11 in]
            n136 = call "Open sequence.vi"("Sequence name"=w286, "error in (no error)"=w287) -> ("User input 1"=w277:T1, "string steps"=w284:string[], "Steps"=w281:T10[], "error out"=w285:errorcluster)  [unwired: 9 in, 1 out]
            n137 = property on="Steps" class="LstBox (strict)"(error in=w285, "Item Names"=w284) -> (error out=w283:errorcluster)  [unwired: 1 in, 1 out]
            n138 = local write "User input 1"(w277) -> ()
            n139 = flat-sequence {
              tunnel: [w303] -> w279
              tunnel: w283 -> [w303]
              tunnel: w281 -> [w302]
              tunnel: [w300] -> w280
              frame #0 {
                w301 = 0
                n140 = Index Array(array=w302, index=w301) -> (element=w300:T10)
                n141 = local write "Steps"(w301) -> ()
              }
            }
            n142 = call "Data step til GUI step.vi"("data step cluster"=w280) -> ("GUI step clluster"=w282:T2)  [unwired: 13 in, 1 out]
            n143 = local write "Step"(w282) -> ()
          }
          event Value Change {
            n144 = event-data() -> ("NewVal"=w315:T2)  [unwired: 1 in, 4 out]
            n145 = feedback #3(0) -> (w306:i32)
            n146 = Increment(x=w306) -> (x+1=w305:i32)
            n147 = feedback-in #3(w305) -> ()
            n148 = call "GUI step til data step.vi"("GUI step clluster"=w315) -> ("data step cluster"=w314:T10)  [unwired: 14 in]
            n149 = local read "Steps"() -> (w316:i32)
            n150 = in-place {
              in-place-border: w314 -> [w322]
              n151 = in-place-array #4(w317, w316) -> ()  [unwired: 1 out]
              n152 = in-place-array #4(w322) -> (w311:T10[])  [unwired: 1 out]
            }
            n153 = local read "User input 1"() -> (w309:T1)
            n154 = Unbundle By Name(w309) -> ("Default value"=w308:dbl)
            n155 = for {
              tunnel: w311 -> [w320] mode=indexing
              tunnel: [w321] -> w310 mode=indexing
              tunnel: w308 -> [w319]
              n156 = call "criteria string.vi"("Sequence step config"=w320, "User input"=w319) -> ("Full criteria string"=w321:string)  [unwired: 12 in, 1 out]
            }
            n157 = property on="Steps" class="LstBox (strict)"(error in=w313, "Item Names"=w310) -> (error out=w312:errorcluster)  [unwired: 1 in, 1 out]
          }
          event "Steps": Value Change {
            n158 = event-data() -> ("OldVal"=w335:i32, "NewVal"=w331:i32)  [unwired: 1 in, 3 out]
            n159 = local read "Step"() -> (w334:T2)
            n160 = call "GUI step til data step.vi"("GUI step clluster"=w334) -> ("data step cluster"=w333:T10)  [unwired: 14 in]
            n161 = in-place {
              in-place-border: w333 -> [w340]
              n162 = in-place-array #5(w332, w335) -> ()  [unwired: 1 out]
              n163 = in-place-array #5(w340) -> (w326:T10[])  [unwired: 1 out]
            }
            n164 = Index Array(array=w326, index=w331) -> (element=w330:T10)
            n165 = local read "User input 1"() -> (w324:T1)
            n166 = call "Data step til GUI step.vi"("data step cluster"=w330) -> ("GUI step clluster"=w329:T2)  [unwired: 13 in, 1 out]
            n167 = local write "Step"(w329) -> ()
            n168 = Unbundle By Name(w324) -> ("Default value"=w323:dbl)
            n169 = for {
              tunnel: w326 -> [w339] mode=indexing
              tunnel: [w338] -> w328 mode=indexing
              tunnel: w323 -> [w337]
              n170 = call "criteria string.vi"("Sequence step config"=w339, "User input"=w337) -> ("Full criteria string"=w338:string)  [unwired: 12 in, 1 out]
            }
            n171 = property on="Steps" class="LstBox (strict)"(error in=w327, "Item Names"=w328) -> (error out=w325:errorcluster)  [unwired: 1 in, 1 out]
          }
          event "Add step": Value Change {
            n172 = event-data() -> ("NewVal"=w345:bool)  [unwired: 1 in, 4 out]
            n173 = case shown="True" w345 {
              tunnel: w344 -> [w348 w352]
              tunnel: [w348 w353] -> w343
              tunnel: w342 -> [w347 w356]
              tunnel: [w347 w351] -> w341
              frame False {
              }
              frame True {
                n174 = local read "User input 1"() -> (w350:T1)
                n175 = Build Array (concatenate)(w356, T10 {"Enabled"=TRUE, "Criteria 1"={"Criteria"=enum."No criteria(True)", "Time or analog value"=0.0, "Primary IO index"=0, "Secondary  IO index"=0, "User_input"=FALSE}, "C1 op C2"=enum."And", "Criteria 2"={"Criteria"=enum."No criteria(True)", "Time or analog value"=0.0, "Primary IO index"=0, "Secondary  IO index"=0, "User_input"=FALSE}, "Action index"=0, "Action Name"="", "Action value"=0.0} ("data step cluster")) -> (w351:T10[])
                n176 = Unbundle By Name(w350) -> ("Default value"=w349:dbl)
                n177 = for {
                  tunnel: w351 -> [w359] mode=indexing
                  tunnel: [w358] -> w354 mode=indexing
                  tunnel: w349 -> [w357]
                  n178 = call "criteria string.vi"("Sequence step config"=w359, "User input"=w357) -> ("Full criteria string"=w358:string)  [unwired: 12 in, 1 out]
                }
                n179 = property on="Steps" class="LstBox (strict)"(error in=w352, "Item Names"=w354) -> (error out=w353:errorcluster)  [unwired: 1 in, 1 out]
              }
            }
          }
          event "Delete step": Value Change {
            n180 = event-data() -> ("NewVal"=w364:bool)  [unwired: 1 in, 4 out]
            n181 = case shown="True" w364 {
              tunnel: w363 -> [w367 w377]
              tunnel: [w367 w378] -> w362
              tunnel: w361 -> [w366 w375]
              tunnel: [w366 w373] -> w360
              frame False {
              }
              frame True {
                n182 = local read "Steps"() -> (w371:i32)
                n183 = Array Size(array=w375) -> (size(s)=w376:i32)
                n184 = case shown="..1" w376 {
                  tunnel: w375 -> [w384 _]
                  tunnel: [w383 w386] -> w373
                  tunnel: w371 -> [w381 _]
                  tunnel: [0 ("Steps") 0 ("Steps")] -> w370
                  frame 2, Default {
                    n185 = Delete From Array(array=w384, length=1, index=w381) -> (array with subset deleted=w383:T10[])  [unwired: 1 out]
                  }
                  frame ..1 {
                    n186 = Build Array(T10 {"Enabled"=TRUE, "Criteria 1"={"Criteria"=enum."No criteria(True)", "Time or analog value"=0.0, "Primary IO index"=0, "Secondary  IO index"=0, "User_input"=FALSE}, "C1 op C2"=enum."Or", "Criteria 2"={"Criteria"=enum."No criteria(True)", "Time or analog value"=0.0, "Primary IO index"=0, "Secondary  IO index"=0, "User_input"=FALSE}, "Action index"=0, "Action Name"="", "Action value"=0.0} ("data step cluster")) -> (w386:T10[])
                  }
                }
                n187 = Index Array(array=w373, index=w370) -> (element=w372:T10)
                n188 = local write "Steps"(w370) -> ()
                n189 = call "Data step til GUI step.vi"("data step cluster"=w372) -> ("GUI step clluster"=w374:T2)  [unwired: 13 in, 1 out]
                n190 = local read "User input 1"() -> (w369:T1)
                n191 = local write "Step"(w374) -> ()
                n192 = Unbundle By Name(w369) -> ("Default value"=w368:dbl)
                n193 = for {
                  tunnel: w373 -> [w390] mode=indexing
                  tunnel: [w389] -> w379 mode=indexing
                  tunnel: w368 -> [w388]
                  n194 = call "criteria string.vi"("Sequence step config"=w390, "User input"=w388) -> ("Full criteria string"=w389:string)  [unwired: 12 in, 1 out]
                }
                n195 = property on="Steps" class="LstBox (strict)"(error in=w377, "Item Names"=w379) -> (error out=w378:errorcluster)  [unwired: 1 in, 1 out]
              }
            }
          }
          event "Move up": Value Change {
            n196 = event-data() -> ("NewVal"=w395:bool)  [unwired: 1 in, 4 out]
            n197 = case shown="True" w395 {
              tunnel: w394 -> [w398 w407]
              tunnel: [w398 w408] -> w393
              tunnel: w392 -> [w397 w403]
              tunnel: [w397 w402] -> w391
              frame False {
              }
              frame True {
                n198 = local read "Steps"() -> (w404:i32)
                n199 = case shown="1, Default" w404 {
                  selector: w404 -> [w410 w414]
                  tunnel: w403 -> [w411 w415]
                  tunnel: [w411 w412] -> w402
                  tunnel: [w410 w413] -> w401
                  frame 0 {
                  }
                  frame 1, Default {
                    n200 = Decrement(x=w414) -> (x-1=w413:i32)
                    n201 = in-place {
                      n202 = in-place-array #6(w415, w414, w413) -> (w417:T10, w416:T10)
                      n203 = in-place-array #6(w416, w417) -> (w412:T10[])  [unwired: 2 out]
                    }
                  }
                }
                n204 = local read "User input 1"() -> (w400:T1)
                n205 = Unbundle By Name(w400) -> ("Default value"=w399:dbl)
                n206 = for {
                  tunnel: w402 -> [w420] mode=indexing
                  tunnel: [w419] -> w409 mode=indexing
                  tunnel: w399 -> [w418]
                  n207 = call "criteria string.vi"("Sequence step config"=w420, "User input"=w418) -> ("Full criteria string"=w419:string)  [unwired: 12 in, 1 out]
                }
                n208 = Index Array(array=w402, index=w401) -> (element=w405:T10)
                n209 = local write "Steps"(w401) -> ()
                n210 = call "Data step til GUI step.vi"("data step cluster"=w405) -> ("GUI step clluster"=w406:T2)  [unwired: 13 in, 1 out]
                n211 = local write "Step"(w406) -> ()
                n212 = property on="Steps" class="LstBox (strict)"(error in=w407, "Item Names"=w409) -> (error out=w408:errorcluster)  [unwired: 1 in, 1 out]
              }
            }
          }
          event "Move down": Value Change {
            n213 = event-data() -> ("NewVal"=w425:bool)  [unwired: 1 in, 4 out]
            n214 = case shown="True" w425 {
              tunnel: w424 -> [w428 w439]
              tunnel: [w428 w440] -> w423
              tunnel: w422 -> [w427 w435]
              tunnel: [w427 w436] -> w421
              frame False {
              }
              frame True {
                n215 = Array Size(array=w435) -> (size(s)=w433:i32)
                n216 = local read "Steps"() -> (w434:i32)
                n217 = Less?(x=w434, y=w433) -> (x < y?=w432:bool)
                n218 = case shown="True" w432 {
                  tunnel: w435 -> [w443 w447]
                  tunnel: [w443 w445] -> w436
                  tunnel: [w442 w446] -> w431
                  tunnel: w434 -> [w442 w444]
                  frame False {
                  }
                  frame True {
                    n219 = Increment(x=w444) -> (x+1=w446:i32)
                    n220 = in-place {
                      n221 = in-place-array #7(w447, w444, w446) -> (w449:T10, w448:T10)
                      n222 = in-place-array #7(w448, w449) -> (w445:T10[])  [unwired: 2 out]
                    }
                  }
                }
                n223 = local read "User input 1"() -> (w430:T1)
                n224 = Unbundle By Name(w430) -> ("Default value"=w429:dbl)
                n225 = for {
                  tunnel: w436 -> [w452] mode=indexing
                  tunnel: [w451] -> w441 mode=indexing
                  tunnel: w429 -> [w450]
                  n226 = call "criteria string.vi"("Sequence step config"=w452, "User input"=w450) -> ("Full criteria string"=w451:string)  [unwired: 12 in, 1 out]
                }
                n227 = Index Array(array=w436, index=w431) -> (element=w437:T10)
                n228 = call "Data step til GUI step.vi"("data step cluster"=w437) -> ("GUI step clluster"=w438:T2)  [unwired: 13 in, 1 out]
                n229 = local write "Steps"(w431) -> ()
                n230 = local write "Step"(w438) -> ()
                n231 = property on="Steps" class="LstBox (strict)"(error in=w439, "Item Names"=w441) -> (error out=w440:errorcluster)  [unwired: 1 in, 1 out]
              }
            }
          }
          event "Help": Value Change {
            n232 = event-data() -> ()  [unwired: 1 in, 5 out]
            n233 = case shown="True" "Help" {
              tunnel: [w459 w461] -> w457
              tunnel: w456 -> [w459 w460]
              frame False {
              }
              frame True {
                n234 = call "Open App Help file.vi"("error In"=w460) -> ("error out"=w461:errorcluster)  [unwired: 14 in]
              }
            }
          }
        }
      }
    }
    frame Error {
      n235 = Unbundle(w467) -> ("code"=w464:i32, "source"=w463:string)  [unwired: 1 out]
      n236 = Format Into String(format string="%d    %s", initial string="Sequence dialog could not be displayed due to error\n\n" ("message"), w464, w463) -> (resulting string=w465:string)  [unwired: 1 in, 1 out]
      n237 = One Button Dialog(message=w465) -> ()  [unwired: 1 in, 1 out]
    }
  }
  "OK" <- w21
  n238 = call "emi_Dialog End.vi"("error in"=w20) -> ("error out"=→"error out":errorcluster)  [unwired: 14 in]
